vi "Update FIFO Drop Statistics.vi"(9 "Header":T1, 10 "FIFO Drop Stat in":u64, 11 "FIFO Drop in":T2) -> (2 "FIFO Drops Stat out":u64, 3 "FIFO Drop out":T2)   [LabVIEW 2021, in "CIFCoreCommon.lvlib"]
uses:
  CIFCoreCommon.lvlib
  Typedef/FIFO Drop Internal Data.ctl
  <vilib>/CIF Foundation/CIF Channels Core/ChannelCommon/typedef/FIFO Header.ctl
  <vilib>/CIF Foundation/CIF Channels Core/ChannelCommon/ChannelCommon.lvlib
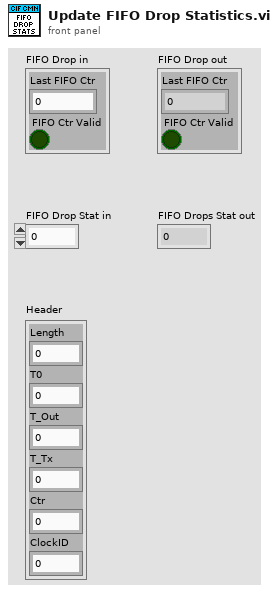
[diagram p1: front panel]
types:
  T1 = typedef "ChannelCommon.lvlib/FIFO Header.ctl" = cluster{"Length":u64, "T0":i64, "T_Out":i64, "T_Tx":i64, "Ctr":u64, "ClockID":u8}
  T2 = typedef "CIFCoreCommon.lvlib/FIFO Drop Internal Data.ctl" = cluster{"Last FIFO Ctr":u64, "FIFO Ctr Valid":bool}
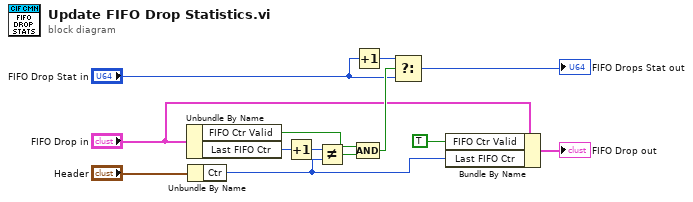
[diagram p0: block diagram]
diagram:
  n1 = Unbundle By Name("FIFO Drop in") -> ("FIFO Ctr Valid"=w12:bool, "Last FIFO Ctr"=w8:u64)
  n2 = Unbundle By Name("Header") -> ("Ctr"=w7:u64)
  n3 = Increment(x=w8) -> (x+1=w6:u64)
  n4 = Not Equal?(x=w6, y=w7) -> (x != y?=w13:bool)
  n5 = Increment(x="FIFO Drop Stat in") -> (x+1=w10:u64)
  n6 = Compound Arithmetic op=AND(w12, w13) -> (w11:bool)
  n7 = Select(t=w10, s=w11, f="FIFO Drop Stat in") -> (s? t:f=→"FIFO Drops Stat out":u64)
  n8 = Bundle By Name(cluster="FIFO Drop in", "FIFO Ctr Valid"=TRUE ("Internal Data.FIFO Ctr Valid"), "Last FIFO Ctr"=w7) -> (→"FIFO Drop out":T2)
